vi "AssertSourceSeparatedFromCompiledCode.vi"(8 "error in":errorcluster, 9 "folders to exclude":string[](array[string]), 10 "search path":path, 11 "TestCase in":refnum<class "TestCase.lvclass">) -> (0 "error out":errorcluster, 3 "TestCase out":refnum<class "TestCase.lvclass">)   [LabVIEW 2017, in "VeriStandTestUtilities.lvlib"]
uses:
  VeriStandTestUtilities.lvlib
  <vilib>/addons/_JKI Toolkits/VI Tester/TestCase.llb/TestCase.lvclass
  <userlib>/_OpenG.lib/file/file.llb/Append Path to Root if Relative - Scalar__ogtk.vi
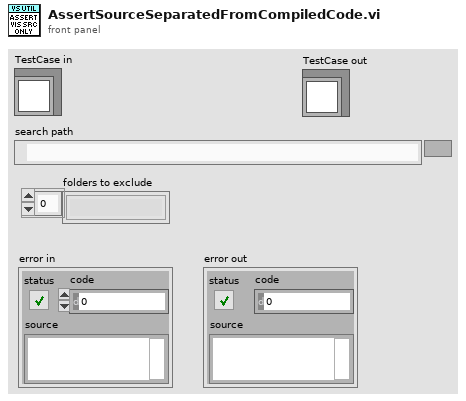
[diagram p1: front panel]
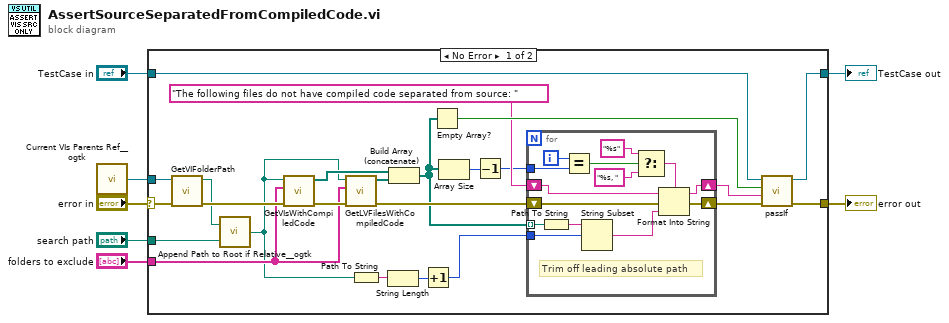
[diagram p0: block diagram]
diagram:
  n1 = call <userlib>:"Current VIs Parents Ref__ogtk.vi"() -> ("Calling VI's Reference"=w1:refnum<vi>)  [unwired: 2 in]
  n2 = case shown="No Error" "error in" {
    selector: "error in" -> [w21 w47]
    tunnel: [w29 w47] -> w7
    tunnel: "search path" -> [w18 _]
    tunnel: "TestCase in" -> [w31 w46]
    tunnel: [w30 w46] -> w3
    tunnel: "folders to exclude" -> [w12 _]
    tunnel: w1 -> [w15 _]
    frame No Error {
      n3 = call "GetVIFolderPath.vi"("error in (no error)"=w21, "VI Reference in"=w15) -> ("error out"=w20:errorcluster, "VI Folder Path out"=w19:path)  [unwired: 8 in]
      n4 = call-poly <userlib>:"Append Path to Root if Relative__ogtk.vi"("Absolute or Relative Path"=w18, "Root Path"=w19) -> ("Absolute or Appended Path"=w8:path)
      n5 = call "GetVIsWithCompiledCode.vi"("error in (no error)"=w20, "Folders to Exclude"=w12, "Search Path"=w8) -> ("error out"=w14:errorcluster, "VIs with compiled code"=w11:path[])  [unwired: 7 in]
      n6 = call "GetLVFilesWithCompiledCode.vi"("error in"=w14, "Folders to Exclude"=w12, "Search Path"=w8) -> ("error out"=w13:errorcluster, "VIs with compiled code"=w10:path[])  [unwired: 7 in]
      n7 = Path To String(path=w8) -> (string=w24:string)
      n8 = String Length(string=w24) -> (length=w23:i32)
      n9 = Build Array (concatenate)(w11, w10) -> (w9:path[])
      n10 = Increment(x=w23) -> (x+1=w22:i32)
      n11 = Empty Array?(array=w9) -> (empty?=w28:bool)
      n12 = Array Size(array=w9) -> (size(s)=w17:i32)
      n13 = Decrement(x=w17) -> (x-1=w16:i32)
      n14 = for {
        tunnel: w9 -> [w36] mode=indexing
        shift-right: [w44] -> w26
        shift-left: "The following files do not have compiled code separated from source: " ("initial string") -> [w45]
        shift-right: [w37] -> w25
        shift-left: w13 -> [w38]
        tunnel: w22 -> [w33]
        tunnel: w16 -> [w32]
        i -> [w43]
        # "Trim off leading absolute path"
        n15 = Path To String(path=w36) -> (string=w35:string)
        n16 = Equal?(x=w43, y=w32) -> (x = y?=w40:bool)
        n17 = String Subset(string=w35, offset (0)=w33) -> (substring=w34:string)  [unwired: 1 in]
        n18 = Select(t="%s" ("format string"), s=w40, f="%s, " ("format string")) -> (s? t:f=w39:string)
        n19 = Format Into String(format string=w39, initial string=w45, error in=w38, w34) -> (resulting string=w44:string, error out=w37:errorcluster)
      }
      n20 = call-dynamic "passIf.vi"("error in (no error)"=w25, "message (\"\")"=w26, "pass"=w28, "TestCase in"=w31) -> ("error out"=w29:errorcluster, "TestCase out"=w30:refnum<class "TestCase.lvclass">)  [unwired: 6 in]
    }
    frame Error {
    }
  }
  "error out" <- w7
  "TestCase out" <- w3
